vi "paramset.vi"(8 "data":u8[](array[numeric]), 10 "byPara":u8) -> (2 "return":i32)   [LabVIEW 2016]
panel:
  in  "cmd_std_header_t":T1
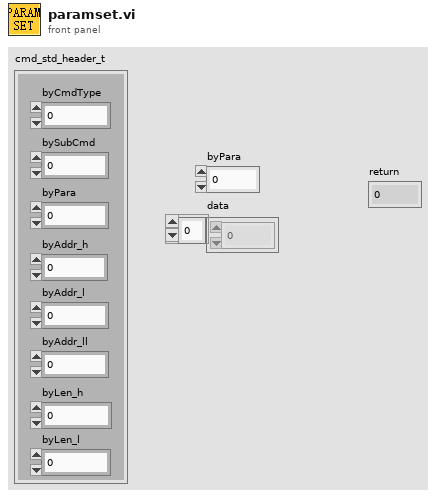
[diagram p1: front panel]
types:
  T1 = cluster{"byCmdType":u8, "bySubCmd":u8, "byPara":u8, "byAddr_h":u8, "byAddr_l":u8, "byAddr_ll":u8, "byLen_h":u8, "byLen_l":u8}
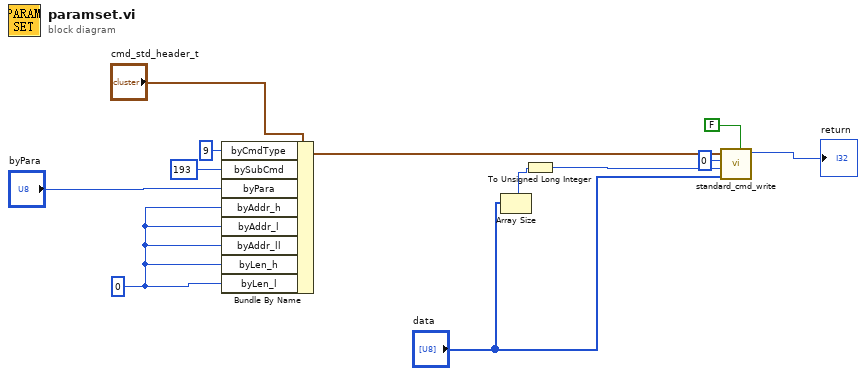
[diagram p0: block diagram]
diagram:
  w3 = u8 0 ("byLen_l")
  n1 = Bundle By Name(cluster="cmd_std_header_t", "byCmdType"=u8 9, "bySubCmd"=u8 193, "byPara"="byPara", "byAddr_h"=w3, "byAddr_l"=w3, "byAddr_ll"=w3, "byLen_h"=w3, "byLen_l"=w3) -> (w11:T1)
  n2 = Array Size(array="data") -> (size(s)=w8:i32)
  n3 = To Unsigned Long Integer(number=w8) -> (unsigned 32bit integer=w7:u32)
  n4 = call "standard_cmd_write.vi"("COM"=FALSE, "data"="data", "dwLen"=w7, "dwAddr"=u32 0, "cmd_std_header_t"=w11) -> ("return"=→"return":i32)  [unwired: 6 in]
